vi "浮点DCBA转换.vi"(11 "数组":i16[](array[numeric]) format="%04xH") -> (3 "数组 2":sgl[](array[numeric]) format="%#.2f")   [LabVIEW 2016, in "数据传输系统-04.lvlib"]
panel:
  # "溶解氧浮点格式采用DCBA"
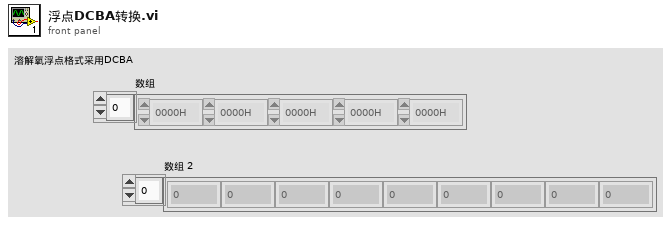
[diagram p1: front panel]
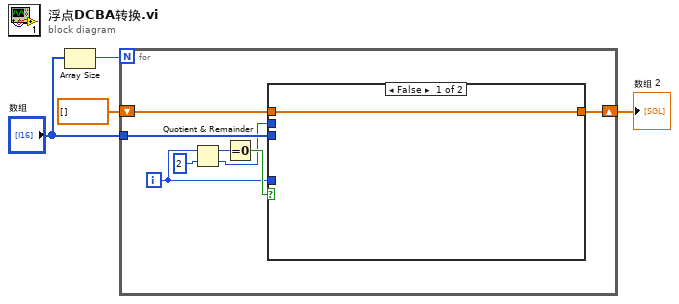
[diagram p0: block diagram]
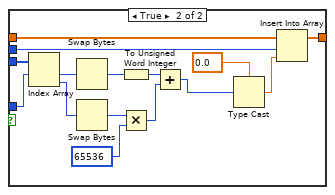
[diagram p2: hidden frame]
diagram:
  n1 = Array Size(array="数组") -> (size(s)=w3:i32)
  n2 = for {
    N: w3 -> [_]
    tunnel: "数组" -> [w10]
    shift-right: [w6] -> w2
    shift-left: sgl[] [] -> [w5]
    i -> [w9]
    n3 = Quotient & Remainder(x=w9, y=2) -> (x-y*floor(x/y)=w7:i32, floor(x/y)=w8:i32)
    n4 = Equal To 0?(x=w7) -> (x = 0?=w11:bool)
    n5 = case shown="False" w11 {
      tunnel: w10 -> [_ w18]
      tunnel: w9 -> [_ w28]
      tunnel: w8 -> [_ w15]
      tunnel: [w13 w16] -> w6
      tunnel: w5 -> [w13 w14]
      frame False {
      }
      frame True {
        n6 = Index Array(array=w18, index #1=w28) -> (element #1=w26:i16, element #2=w25:i16)  [unwired: 1 in]
        n7 = Swap Bytes(anything=w26) -> (byte swapped=w21:i16)
        n8 = Swap Bytes(anything=w25) -> (byte swapped=w24:i16)
        n9 = To Unsigned Word Integer(number=w21) -> (unsigned 16bit integer=w20:u16)
        n10 = Multiply(x=w24, y=u32 65536) -> (x*y=w22:u32)
        n11 = Add ("加")(x=w20, y=w22) -> (x+y=w19:u32)
        n12 = Type Cast(type=sgl 0.0, x=w19) -> (*(type *) &x=w17:sgl)
        n13 = Insert Into Array(array=w14, index=w15, new element=w17) -> (w16:sgl[])
      }
    }
  }
  "数组 2" <- w2
